vi "Read TriggerModulo.vi"(8 "error in (no error)":errorcluster, 11 "BME_DG_Chnl in":refnum<class "BME_DG_Chnl.lvclass">) -> (0 "error out":errorcluster, 2 "TriggerModulo":i32, 3 "BME_DG_Chnl out":refnum<class "BME_DG_Chnl.lvclass">)   [LabVIEW 2009, in "POLARIS BME DG.lvlib" / "BME_DG_Chnl.lvclass"]
uses:
  BME_DG_Chnl.lvclass
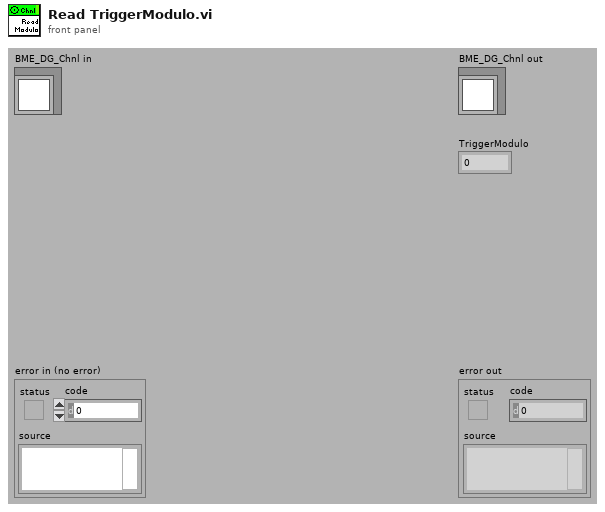
[diagram p1: front panel]
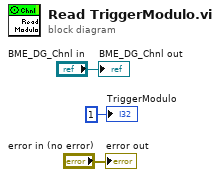
[diagram p0: block diagram]
diagram:
  "error out" <- "error in (no error)"
  "BME_DG_Chnl out" <- "BME_DG_Chnl in"
  "TriggerModulo" <- 1 ("Numeric")
